vi "Reset Unit.vi"(8 "error in (no error)":errorcluster, 11 "Ethernet in":refnum<class "ENET_BS1201.lvclass">) -> (0 "error out":errorcluster, 3 "Ethernet out":refnum<class "ENET_BS1201.lvclass">)   [LabVIEW 2021, in "BS120x Driver.lvlib" / "ENET_BS1201.lvclass"]
uses:
  ENET_BS1201.lvclass
  C:/Users/Public/Documents/Projects/7100-00109 SW BS1201 LV Driver/trunk/source/ENET_BS120x/ENET_BS120x.lvclass
  ENET_BS120x/ENET_BS120x.lvclass
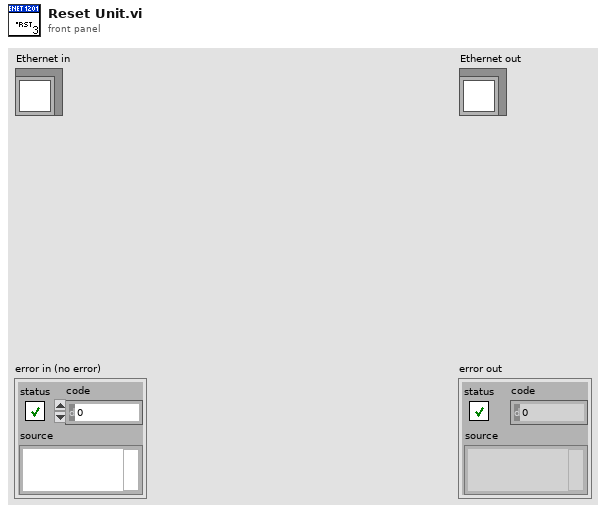
[diagram p1: front panel]
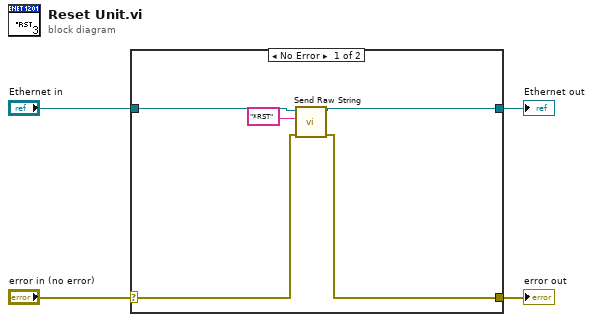
[diagram p0: block diagram]
diagram:
  n1 = case shown="No Error" "error in (no error)" {
    selector: "error in (no error)" -> [w6 w11]
    tunnel: [w5 w11] -> w3
    tunnel: [w8 w10] -> w1
    tunnel: "Ethernet in" -> [w9 w10]
    frame No Error {
      n2 = call "Send Raw String.vi"("error in (no error)"=w6, "String Data"="*RST", "ENET in"=w9) -> ("error out"=w5:errorcluster, "ENET out"=w8:refnum<class "ENET_BS1201.lvclass">)  [unwired: 7 in]
    }
    frame Error {
    }
  }
  "error out" <- w3
  "Ethernet out" <- w1
